vi "Stephan-Test connect power meter.vi"() -> ()   [LabVIEW 2018]
panel:
  out "Power":dbl
  in  "Ratio (R/T)":dbl=0.01865
  in  "error in (no error) 2":errorcluster caption="error in (no error)" {"code" format="%.0x"}
  in  "Average Count":i32=10 min=1 step=1
  in  "Wavelength [nm]":dbl=930.0 caption="Wavelength (0.0)"
  in  "Avg. Time (0.0) [sec.]":dbl=0.1 caption="Average Time (0.0)" min=0.1 max=5.0 step=0.1
  out "Average Count 2":i32 caption="Average Time"
  out "Avg. Time  [sec.]":dbl caption="Average Time"
  out "Wavelength [nm] 2":dbl caption="Wavelength"
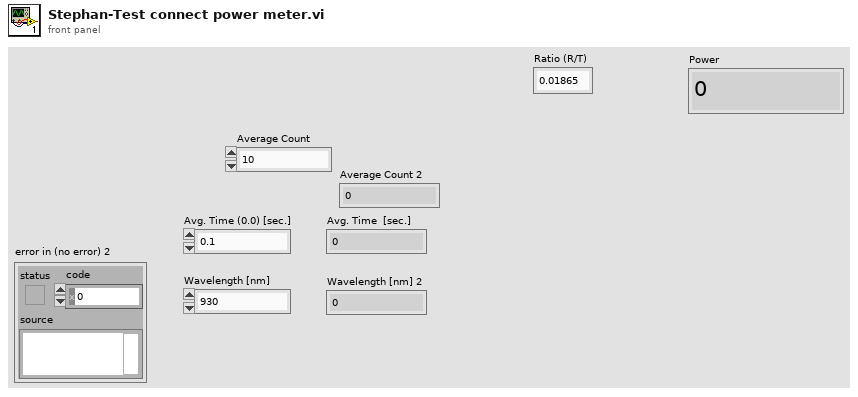
[diagram p1: front panel]
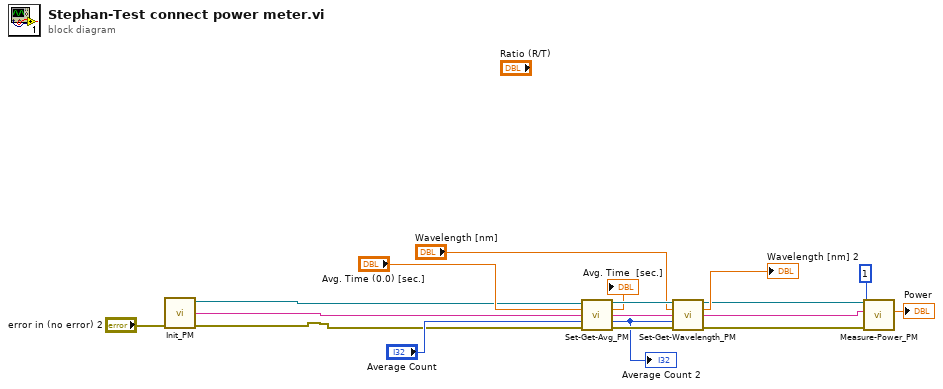
[diagram p0: block diagram]
diagram:
  n1 = call "Init_PM.vi"("error in (no error)"="error in (no error) 2") -> ("error out"=w6:errorcluster, "Sensor Name"=w7:string, "instrument handle out"=w8:refnum<visa-resource-name>)  [unwired: 8 in]
  n2 = call "Set-Get-Avg_PM.vi"("instrument handle"=w8, "Average Time (0.0)"="Avg. Time (0.0) [sec.]", "Sensor"=w7, "Average Count"="Average Count", "error in (no error)"=w6) -> ("instrument handle out"=w16:refnum<visa-resource-name>, "Average Time"=→"Avg. Time  [sec.]":dbl, "Sensor 2"=w14:string, "Average Count"=w13:i32, "error out"=w17:errorcluster)  [unwired: 6 in]
  "Average Count 2" <- w13
  n3 = call "Set-Get-Wavelength_PM.vi"("instrument handle"=w16, "Wavelength"="Wavelength [nm]", "Sensor Name"=w14, "Average Count"=w13, "error in (no error)"=w17) -> ("instrument handle out"=w5:refnum<visa-resource-name>, "Wavelength"=→"Wavelength [nm] 2":dbl, "Sensor Name 2"=w4:string, "error out"=w3:errorcluster)  [unwired: 6 in, 1 out]
  n4 = call "Measure-Power_PM.vi"("error in (no error)"=w3, "Numeric"=1, "Sensor"=w4, "instrument handle"=w5) -> ("Power"=→"Power":dbl)  [unwired: 5 in, 2 out]
